vi "Start.vi"(8 "error in (no error)":errorcluster, 11 "bt_System in":refnum<class "bt_System.lvclass">) -> (0 "error out":errorcluster, 3 "bt_System out":refnum<class "bt_System.lvclass">)   [LabVIEW 2021, in "BT.lvlib" / "bt_System.lvclass"]
uses:
  bt_System.lvclass
  bt_System.lvclass/bt_System.ctl
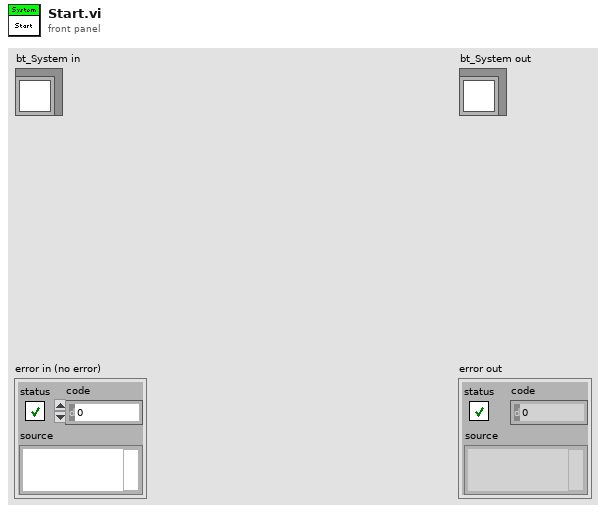
[diagram p1: front panel]
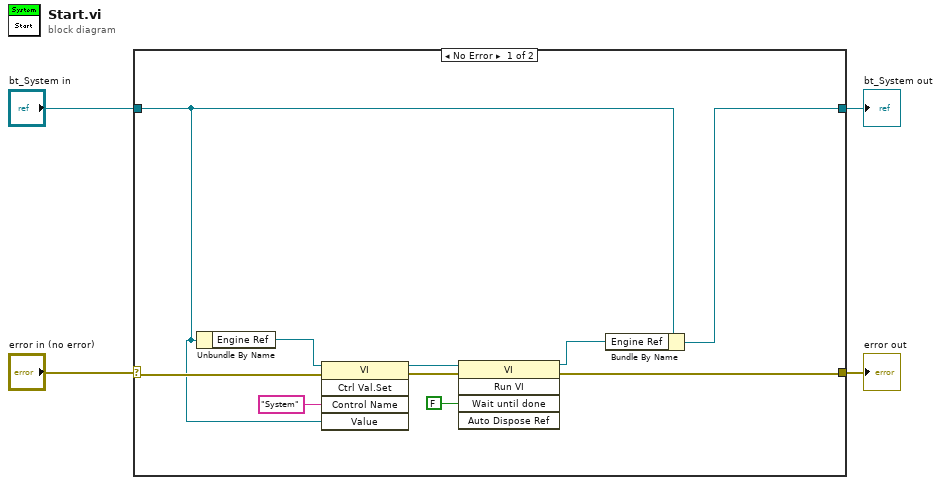
[diagram p0: block diagram]
diagram:
  n1 = case shown="No Error" "error in (no error)" {
    selector: "error in (no error)" -> [w10 w16]
    tunnel: [w14 w16] -> w3
    tunnel: [w12 w15] -> w1
    tunnel: "bt_System in" -> [w7 w15]
    frame No Error {
      n2 = Unbundle By Name(w7) -> ("Engine Ref"=w11:refnum<vi>)
      n3 = invoke class="VI" method="Ctrl Val.Set"(reference=w11, error in=w10, "Control Name"="System", "Value"=w7) -> (reference out=w9:refnum<vi>, error out=w8:errorcluster)  [unwired: 1 in, 3 out]
      n4 = invoke class="VI" method="Run VI"(reference=w9, error in=w8, "Wait until done"=FALSE ("Wait Until Done")) -> (reference out=w13:refnum<vi>, error out=w14:errorcluster)  [unwired: 2 in, 3 out]
      n5 = Bundle By Name(cluster=w7, "Engine Ref"=w13) -> (w12:refnum<class "bt_System.lvclass">)
    }
    frame Error {
    }
  }
  "error out" <- w3
  "bt_System out" <- w1
